vi "multi-function-fpga.vi"() -> ()   [LabVIEW 2016]
uses:
  <vilib>/rvi/Emulation/niFpgaGetClockAttributes.vi
  <vilib>/rvi/Emulation/niFpgaSctlEmulationGetInTimedLoop.vi
  <vilib>/rvi/Emulation/niFpgaEmulationReportErrorSimple.vi
  <vilib>/rvi/eio/common/nirviEmuTemplateMethod_errors.vi
  <vilib>/rvi/Emulation/niFpgaCriticalErrorInLSC.vi
  <vilib>/eio/EIONode/EIONode.xnode
panel:
  in  "and1":fxp<+/-,20,5>=3.5 format="%#_17g"
  in  "or15":fxp<+/-,20,5>=3.5 format="%#_17g"
  in  "or14":fxp<+/-,20,5>=3.5 format="%#_17g"
  in  "or13":fxp<+/-,20,5>=3.5 format="%#_17g"
  in  "or12":fxp<+/-,20,5>=3.5 format="%#_17g"
  in  "or11":fxp<+/-,20,5>=3.5 format="%#_17g"
  in  "or10":fxp<+/-,20,5>=3.5 format="%#_17g"
  in  "or9":fxp<+/-,20,5>=3.5 format="%#_17g"
  in  "or8":fxp<+/-,20,5>=3.5 format="%#_17g"
  in  "or7":fxp<+/-,20,5>=3.5 format="%#_17g"
  in  "or6":fxp<+/-,20,5>=3.5 format="%#_17g"
  in  "or5":fxp<+/-,20,5>=3.5 format="%#_17g"
  in  "or4":fxp<+/-,20,5>=3.5 format="%#_17g"
  in  "or3":fxp<+/-,20,5>=3.5 format="%#_17g"
  in  "or2":fxp<+/-,20,5>=3.5 format="%#_17g"
  in  "or1":fxp<+/-,20,5>=3.5 format="%#_17g"
  in  "or0":fxp<+/-,20,5>=3.5 format="%#_17g"
  in  "and15":fxp<+/-,20,5>=3.5 format="%#_17g"
  in  "and14":fxp<+/-,20,5>=3.5 format="%#_17g"
  in  "and13":fxp<+/-,20,5>=3.5 format="%#_17g"
  in  "and12":fxp<+/-,20,5>=3.5 format="%#_17g"
  in  "and11":fxp<+/-,20,5>=3.5 format="%#_17g"
  in  "and10":fxp<+/-,20,5>=3.5 format="%#_17g"
  in  "and9":fxp<+/-,20,5>=3.5 format="%#_17g"
  in  "and8":fxp<+/-,20,5>=3.5 format="%#_17g"
  in  "and7":fxp<+/-,20,5>=3.5 format="%#_17g"
  in  "and6":fxp<+/-,20,5>=3.5 format="%#_17g"
  in  "and5":fxp<+/-,20,5>=3.5 format="%#_17g"
  in  "and4":fxp<+/-,20,5>=3.5 format="%#_17g"
  in  "and3":fxp<+/-,20,5>=3.5 format="%#_17g"
  in  "and2":fxp<+/-,20,5>=3.5 format="%#_17g"
  in  "and0":fxp<+/-,20,5>=3.5 format="%#_17g"
  in  "s15":fxp<+/-,20,5>=3.5 format="%#_17g"
  in  "s14":fxp<+/-,20,5>=3.5 format="%#_17g"
  in  "s13":fxp<+/-,20,5>=3.5 format="%#_17g"
  in  "s12":fxp<+/-,20,5>=3.5 format="%#_17g"
  in  "s11":fxp<+/-,20,5>=3.5 format="%#_17g"
  in  "s10":fxp<+/-,20,5>=3.5 format="%#_17g"
  in  "s9":fxp<+/-,20,5>=3.5 format="%#_17g"
  in  "s8":fxp<+/-,20,5>=3.5 format="%#_17g"
  in  "s7":fxp<+/-,20,5>=3.5 format="%#_17g"
  in  "s6":fxp<+/-,20,5>=3.5 format="%#_17g"
  in  "s5":fxp<+/-,20,5>=3.5 format="%#_17g"
  in  "s4":fxp<+/-,20,5>=3.5 format="%#_17g"
  in  "s3":fxp<+/-,20,5>=3.5 format="%#_17g"
  in  "s2":fxp<+/-,20,5>=3.5 format="%#_17g"
  in  "s1":fxp<+/-,20,5>=3.5 format="%#_17g"
  in  "s0":fxp<+/-,20,5>=3.5 format="%#_17g"
  out "Mod2/DIO24":bool
  in  "OUT12":T1(ring)
  in  "iter12":fxp<+/-,20,5> format="%#_17g"
  out "Mod2/DIO26":bool
  in  "OUT13":T1(ring)
  in  "iter13":fxp<+/-,20,5> format="%#_17g"
  out "Mod2/DIO28":bool
  in  "OUT14":T1(ring)
  in  "iter14":fxp<+/-,20,5> format="%#_17g"
  out "Mod2/DIO30":bool
  in  "OUT15":T1(ring)
  in  "iter15":fxp<+/-,20,5> format="%#_17g"
  out "Mod2/DIO16":bool
  in  "OUT8":T1(ring)
  in  "iter8":fxp<+/-,20,5> format="%#_17g"
  out "Mod2/DIO18":bool
  in  "OUT9":T1(ring)
  in  "iter9":fxp<+/-,20,5> format="%#_17g"
  out "Mod2/DIO20":bool
  in  "OUT10":T1(ring)
  in  "iter10":fxp<+/-,20,5> format="%#_17g"
  out "Mod2/DIO22":bool
  in  "OUT11":T1(ring)
  in  "iter11":fxp<+/-,20,5> format="%#_17g"
  out "Mod2/DIO8":bool
  in  "OUT4":T1(ring)
  in  "iter4":fxp<+/-,20,5> format="%#_17g"
  out "Mod2/DIO10":bool
  in  "OUT5":T1(ring)
  in  "iter5":fxp<+/-,20,5> format="%#_17g"
  out "Mod2/DIO12":bool
  in  "OUT6":T1(ring)
  in  "iter6":fxp<+/-,20,5> format="%#_17g"
  out "Mod2/DIO14":bool
  in  "OUT7":T1(ring)
  in  "iter7":fxp<+/-,20,5> format="%#_17g"
  out "Mod2/DIO0":bool
  in  "OUT0":T1(ring)
  in  "iter0":fxp<+/-,20,5> format="%#_17g"
  out "Mod2/DIO2":bool
  in  "OUT1":T1(ring)
  in  "iter1":fxp<+/-,20,5> format="%#_17g"
  out "Mod2/DIO4":bool
  in  "OUT2":T1(ring)
  in  "iter2":fxp<+/-,20,5> format="%#_17g"
  out "Mod2/DIO6":bool
  in  "iter3":fxp<+/-,20,5> format="%#_17g"
  in  "OUT3":T1(ring)
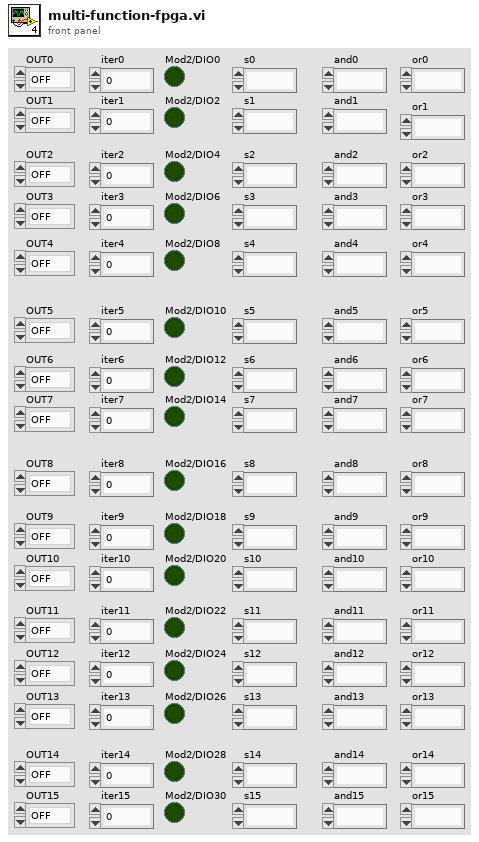
[diagram p1: front panel]
types:
  T1 = enum16{"OFF", "SWITCH", "AND GATE", "OR GATE", "ITERATION"}
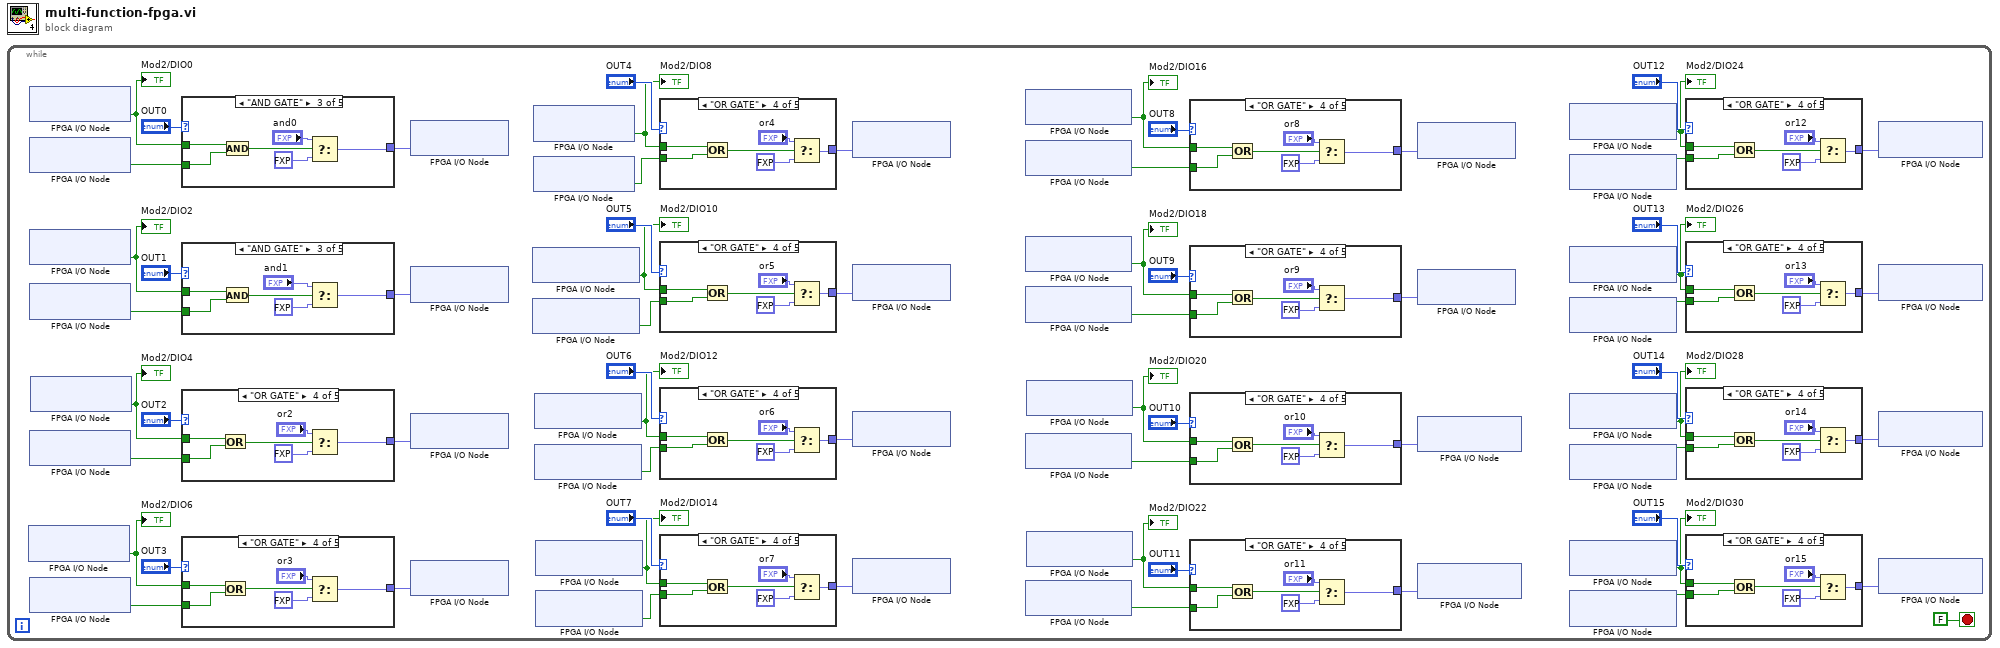
[diagram p0: block diagram]
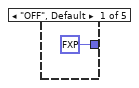
[diagram p2: hidden frame]
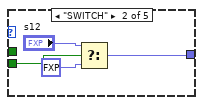
[diagram p3: hidden frame]
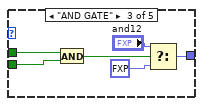
[diagram p4: hidden frame]
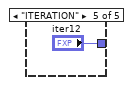
[diagram p5: hidden frame]
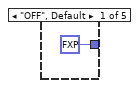
[diagram p6: hidden frame]
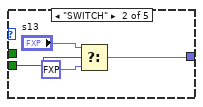
[diagram p7: hidden frame]
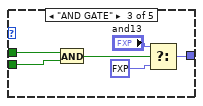
[diagram p8: hidden frame]
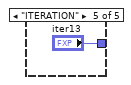
[diagram p9: hidden frame]
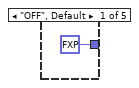
[diagram p10: hidden frame]
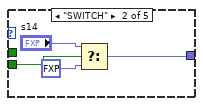
[diagram p11: hidden frame]
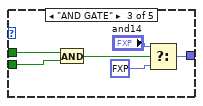
[diagram p12: hidden frame]
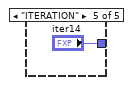
[diagram p13: hidden frame]
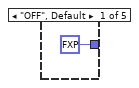
[diagram p14: hidden frame]
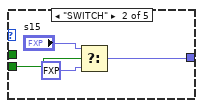
[diagram p15: hidden frame]
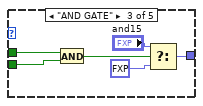
[diagram p16: hidden frame]
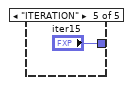
[diagram p17: hidden frame]
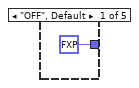
[diagram p18: hidden frame]
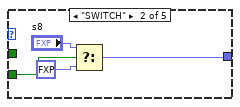
[diagram p19: hidden frame]
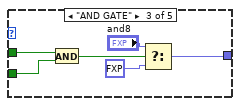
[diagram p20: hidden frame]
diagram:
  n1 = while {
    stop <- FALSE stop-if-true
    n2 = xnode "FPGA I/O Node"() -> ("Mod2/DIO6"=w62:bool)  [unwired: 1 in, 1 out]
    "Mod2/DIO6" <- w62
    n3 = xnode "FPGA I/O Node"() -> ("Mod2/DIO0"=w50:bool)  [unwired: 1 in, 1 out]
    "Mod2/DIO0" <- w50
    n4 = xnode "FPGA I/O Node"() -> ("Mod2/DIO1"=w51:bool)  [unwired: 1 in, 1 out]
    n5 = xnode "FPGA I/O Node"() -> ("Mod2/DIO2"=w54:bool)  [unwired: 1 in, 1 out]
    "Mod2/DIO2" <- w54
    n6 = xnode "FPGA I/O Node"() -> ("Mod2/DIO3"=w55:bool)  [unwired: 1 in, 1 out]
    n7 = xnode "FPGA I/O Node"() -> ("Mod2/DIO5"=w59:bool)  [unwired: 1 in, 1 out]
    n8 = xnode "FPGA I/O Node"() -> ("Mod2/DIO7"=w64:bool)  [unwired: 1 in, 1 out]
    n9 = xnode "FPGA I/O Node"() -> ("Mod2/DIO4"=w58:bool)  [unwired: 1 in, 1 out]
    "Mod2/DIO4" <- w58
    n10 = case shown="\"AND GATE\"" "OUT0" {
      tunnel: w51 -> [_ w286 w291 w297 _]
      tunnel: w50 -> [_ _ w292 w298 _]
      tunnel: [fxp<+/-,20,5> 0.0 ("Mod4/AO0") w283 w287 w293 "iter0"] -> w49
      frame "OFF", Default {
      }
      frame "SWITCH" {
        n11 = Select(t="s0", s=w286, f=fxp<+/-,20,5> 0.0 ("Mod4/AO0")) -> (s? t:f=w283:fxp<+/-,20,5>)
      }
      frame "AND GATE" {
        n12 = And(x=w292, y=w291) -> (x .and. y?=w288:bool)
        n13 = Select(t="and0", s=w288, f=fxp<+/-,20,5> 0.0 ("Mod4/AO0")) -> (s? t:f=w287:fxp<+/-,20,5>)
      }
      frame "OR GATE" {
        n14 = Or(x=w298, y=w297) -> (x .or. y?=w296:bool)
        n15 = Select(t="or0", s=w296, f=fxp<+/-,20,5> 0.0 ("Mod4/AO0")) -> (s? t:f=w293:fxp<+/-,20,5>)
      }
      frame "ITERATION" {
      }
    }
    n16 = case shown="\"AND GATE\"" "OUT1" {
      tunnel: w55 -> [_ w304 w309 w315 _]
      tunnel: w54 -> [_ _ w310 w316 _]
      tunnel: [fxp<+/-,20,5> 0.0 ("Mod4/AO0") w301 w305 w311 "iter1"] -> w53
      frame "OFF", Default {
      }
      frame "SWITCH" {
        n17 = Select(t="s1", s=w304, f=fxp<+/-,20,5> 0.0 ("Mod4/AO0")) -> (s? t:f=w301:fxp<+/-,20,5>)
      }
      frame "AND GATE" {
        n18 = And(x=w310, y=w309) -> (x .and. y?=w306:bool)
        n19 = Select(t="and1", s=w306, f=fxp<+/-,20,5> 0.0 ("Mod4/AO0")) -> (s? t:f=w305:fxp<+/-,20,5>)
      }
      frame "OR GATE" {
        n20 = Or(x=w316, y=w315) -> (x .or. y?=w314:bool)
        n21 = Select(t="or1", s=w314, f=fxp<+/-,20,5> 0.0 ("Mod4/AO0")) -> (s? t:f=w311:fxp<+/-,20,5>)
      }
      frame "ITERATION" {
      }
    }
    n22 = case shown="\"OR GATE\"" "OUT2" {
      tunnel: w59 -> [_ w322 w327 w333 _]
      tunnel: w58 -> [_ _ w328 w334 _]
      tunnel: [fxp<+/-,20,5> 0.0 ("Mod4/AO0") w319 w323 w329 "iter2"] -> w57
      frame "OFF", Default {
      }
      frame "SWITCH" {
        n23 = Select(t="s2", s=w322, f=fxp<+/-,20,5> 0.0 ("Mod4/AO0")) -> (s? t:f=w319:fxp<+/-,20,5>)
      }
      frame "AND GATE" {
        n24 = And(x=w328, y=w327) -> (x .and. y?=w324:bool)
        n25 = Select(t="and2", s=w324, f=fxp<+/-,20,5> 0.0 ("Mod4/AO0")) -> (s? t:f=w323:fxp<+/-,20,5>)
      }
      frame "OR GATE" {
        n26 = Or(x=w334, y=w333) -> (x .or. y?=w332:bool)
        n27 = Select(t="or2", s=w332, f=fxp<+/-,20,5> 0.0 ("Mod4/AO0")) -> (s? t:f=w329:fxp<+/-,20,5>)
      }
      frame "ITERATION" {
      }
    }
    n28 = case shown="\"OR GATE\"" "OUT3" {
      tunnel: w64 -> [_ w340 w345 w351 _]
      tunnel: w62 -> [_ _ w346 w352 _]
      tunnel: [fxp<+/-,20,5> 0.0 ("Mod4/AO0") w337 w341 w347 "iter3"] -> w61
      frame "OFF", Default {
      }
      frame "SWITCH" {
        n29 = Select(t="s3", s=w340, f=fxp<+/-,20,5> 0.0 ("Mod4/AO0")) -> (s? t:f=w337:fxp<+/-,20,5>)
      }
      frame "AND GATE" {
        n30 = And(x=w346, y=w345) -> (x .and. y?=w342:bool)
        n31 = Select(t="and3", s=w342, f=fxp<+/-,20,5> 0.0 ("Mod4/AO0")) -> (s? t:f=w341:fxp<+/-,20,5>)
      }
      frame "OR GATE" {
        n32 = Or(x=w352, y=w351) -> (x .or. y?=w350:bool)
        n33 = Select(t="or3", s=w350, f=fxp<+/-,20,5> 0.0 ("Mod4/AO0")) -> (s? t:f=w347:fxp<+/-,20,5>)
      }
      frame "ITERATION" {
      }
    }
    n34 = xnode "FPGA I/O Node"("Mod4/AO0"=w49) -> ()  [unwired: 1 in, 1 out]
    n35 = xnode "FPGA I/O Node"("Mod4/AO1"=w53) -> ()  [unwired: 1 in, 1 out]
    n36 = xnode "FPGA I/O Node"("Mod4/AO2"=w57) -> ()  [unwired: 1 in, 1 out]
    n37 = xnode "FPGA I/O Node"("Mod4/AO3"=w61) -> ()  [unwired: 1 in, 1 out]
    n38 = xnode "FPGA I/O Node"() -> ("Mod2/DIO10"=w38:bool)  [unwired: 1 in, 1 out]
    "Mod2/DIO10" <- w38
    n39 = xnode "FPGA I/O Node"() -> ("Mod2/DIO11"=w39:bool)  [unwired: 1 in, 1 out]
    n40 = xnode "FPGA I/O Node"() -> ("Mod2/DIO8"=w34:bool)  [unwired: 1 in, 1 out]
    "Mod2/DIO8" <- w34
    n41 = xnode "FPGA I/O Node"() -> ("Mod2/DIO9"=w35:bool)  [unwired: 1 in, 1 out]
    n42 = xnode "FPGA I/O Node"() -> ("Mod2/DIO12"=w42:bool)  [unwired: 1 in, 1 out]
    "Mod2/DIO12" <- w42
    n43 = xnode "FPGA I/O Node"() -> ("Mod2/DIO13"=w43:bool)  [unwired: 1 in, 1 out]
    n44 = xnode "FPGA I/O Node"() -> ("Mod2/DIO14"=w46:bool)  [unwired: 1 in, 1 out]
    "Mod2/DIO14" <- w46
    n45 = xnode "FPGA I/O Node"() -> ("Mod2/DIO15"=w47:bool)  [unwired: 1 in, 1 out]
    n46 = case shown="\"OR GATE\"" "OUT4" {
      tunnel: w35 -> [_ w214 w219 w225 _]
      tunnel: w34 -> [_ _ w220 w226 _]
      tunnel: [fxp<+/-,20,5> 0.0 ("Mod4/AO0") w211 w215 w221 "iter4"] -> w33
      frame "OFF", Default {
      }
      frame "SWITCH" {
        n47 = Select(t="s4", s=w214, f=fxp<+/-,20,5> 0.0 ("Mod4/AO0")) -> (s? t:f=w211:fxp<+/-,20,5>)
      }
      frame "AND GATE" {
        n48 = And(x=w220, y=w219) -> (x .and. y?=w216:bool)
        n49 = Select(t="and4", s=w216, f=fxp<+/-,20,5> 0.0 ("Mod4/AO0")) -> (s? t:f=w215:fxp<+/-,20,5>)
      }
      frame "OR GATE" {
        n50 = Or(x=w226, y=w225) -> (x .or. y?=w224:bool)
        n51 = Select(t="or4", s=w224, f=fxp<+/-,20,5> 0.0 ("Mod4/AO0")) -> (s? t:f=w221:fxp<+/-,20,5>)
      }
      frame "ITERATION" {
      }
    }
    n52 = case shown="\"OR GATE\"" "OUT5" {
      tunnel: w39 -> [_ w232 w237 w243 _]
      tunnel: w38 -> [_ _ w238 w244 _]
      tunnel: [fxp<+/-,20,5> 0.0 ("Mod4/AO0") w229 w233 w239 "iter5"] -> w37
      frame "OFF", Default {
      }
      frame "SWITCH" {
        n53 = Select(t="s5", s=w232, f=fxp<+/-,20,5> 0.0 ("Mod4/AO0")) -> (s? t:f=w229:fxp<+/-,20,5>)
      }
      frame "AND GATE" {
        n54 = And(x=w238, y=w237) -> (x .and. y?=w234:bool)
        n55 = Select(t="and5", s=w234, f=fxp<+/-,20,5> 0.0 ("Mod4/AO0")) -> (s? t:f=w233:fxp<+/-,20,5>)
      }
      frame "OR GATE" {
        n56 = Or(x=w244, y=w243) -> (x .or. y?=w242:bool)
        n57 = Select(t="or5", s=w242, f=fxp<+/-,20,5> 0.0 ("Mod4/AO0")) -> (s? t:f=w239:fxp<+/-,20,5>)
      }
      frame "ITERATION" {
      }
    }
    n58 = case shown="\"OR GATE\"" "OUT6" {
      tunnel: w43 -> [_ w250 w255 w261 _]
      tunnel: w42 -> [_ _ w256 w262 _]
      tunnel: [fxp<+/-,20,5> 0.0 ("Mod4/AO0") w247 w251 w257 "iter6"] -> w41
      frame "OFF", Default {
      }
      frame "SWITCH" {
        n59 = Select(t="s6", s=w250, f=fxp<+/-,20,5> 0.0 ("Mod4/AO0")) -> (s? t:f=w247:fxp<+/-,20,5>)
      }
      frame "AND GATE" {
        n60 = And(x=w256, y=w255) -> (x .and. y?=w252:bool)
        n61 = Select(t="and6", s=w252, f=fxp<+/-,20,5> 0.0 ("Mod4/AO0")) -> (s? t:f=w251:fxp<+/-,20,5>)
      }
      frame "OR GATE" {
        n62 = Or(x=w262, y=w261) -> (x .or. y?=w260:bool)
        n63 = Select(t="or6", s=w260, f=fxp<+/-,20,5> 0.0 ("Mod4/AO0")) -> (s? t:f=w257:fxp<+/-,20,5>)
      }
      frame "ITERATION" {
      }
    }
    n64 = case shown="\"OR GATE\"" "OUT7" {
      tunnel: w47 -> [_ w268 w273 w279 _]
      tunnel: w46 -> [_ _ w274 w280 _]
      tunnel: [fxp<+/-,20,5> 0.0 ("Mod4/AO0") w265 w269 w275 "iter7"] -> w45
      frame "OFF", Default {
      }
      frame "SWITCH" {
        n65 = Select(t="s7", s=w268, f=fxp<+/-,20,5> 0.0 ("Mod4/AO0")) -> (s? t:f=w265:fxp<+/-,20,5>)
      }
      frame "AND GATE" {
        n66 = And(x=w274, y=w273) -> (x .and. y?=w270:bool)
        n67 = Select(t="and7", s=w270, f=fxp<+/-,20,5> 0.0 ("Mod4/AO0")) -> (s? t:f=w269:fxp<+/-,20,5>)
      }
      frame "OR GATE" {
        n68 = Or(x=w280, y=w279) -> (x .or. y?=w278:bool)
        n69 = Select(t="or7", s=w278, f=fxp<+/-,20,5> 0.0 ("Mod4/AO0")) -> (s? t:f=w275:fxp<+/-,20,5>)
      }
      frame "ITERATION" {
      }
    }
    n70 = xnode "FPGA I/O Node"("Mod4/AO4"=w33) -> ()  [unwired: 1 in, 1 out]
    n71 = xnode "FPGA I/O Node"("Mod4/AO5"=w37) -> ()  [unwired: 1 in, 1 out]
    n72 = xnode "FPGA I/O Node"("Mod4/AO6"=w41) -> ()  [unwired: 1 in, 1 out]
    n73 = xnode "FPGA I/O Node"("Mod4/AO7"=w45) -> ()  [unwired: 1 in, 1 out]
    n74 = xnode "FPGA I/O Node"() -> ("Mod2/DIO16"=w18:bool)  [unwired: 1 in, 1 out]
    "Mod2/DIO16" <- w18
    n75 = xnode "FPGA I/O Node"() -> ("Mod2/DIO17"=w19:bool)  [unwired: 1 in, 1 out]
    n76 = xnode "FPGA I/O Node"() -> ("Mod2/DIO18"=w22:bool)  [unwired: 1 in, 1 out]
    "Mod2/DIO18" <- w22
    n77 = xnode "FPGA I/O Node"() -> ("Mod2/DIO19"=w23:bool)  [unwired: 1 in, 1 out]
    n78 = xnode "FPGA I/O Node"() -> ("Mod2/DIO21"=w27:bool)  [unwired: 1 in, 1 out]
    n79 = xnode "FPGA I/O Node"() -> ("Mod2/DIO23"=w31:bool)  [unwired: 1 in, 1 out]
    n80 = xnode "FPGA I/O Node"() -> ("Mod2/DIO20"=w26:bool)  [unwired: 1 in, 1 out]
    "Mod2/DIO20" <- w26
    n81 = xnode "FPGA I/O Node"() -> ("Mod2/DIO22"=w30:bool)  [unwired: 1 in, 1 out]
    "Mod2/DIO22" <- w30
    n82 = case shown="\"OR GATE\"" "OUT8" {
      tunnel: w19 -> [_ w142 w147 w153 _]
      tunnel: w18 -> [_ _ w148 w154 _]
      tunnel: [fxp<+/-,20,5> 0.0 ("Mod4/AO0") w139 w143 w149 "iter8"] -> w17
      frame "OFF", Default {
      }
      frame "SWITCH" {
        n83 = Select(t="s8", s=w142, f=fxp<+/-,20,5> 0.0 ("Mod4/AO0")) -> (s? t:f=w139:fxp<+/-,20,5>)
      }
      frame "AND GATE" {
        n84 = And(x=w148, y=w147) -> (x .and. y?=w144:bool)
        n85 = Select(t="and8", s=w144, f=fxp<+/-,20,5> 0.0 ("Mod4/AO0")) -> (s? t:f=w143:fxp<+/-,20,5>)
      }
      frame "OR GATE" {
        n86 = Or(x=w154, y=w153) -> (x .or. y?=w152:bool)
        n87 = Select(t="or8", s=w152, f=fxp<+/-,20,5> 0.0 ("Mod4/AO0")) -> (s? t:f=w149:fxp<+/-,20,5>)
      }
      frame "ITERATION" {
      }
    }
    n88 = case shown="\"OR GATE\"" "OUT9" {
      tunnel: w23 -> [_ w160 w165 w171 _]
      tunnel: w22 -> [_ _ w166 w172 _]
      tunnel: [fxp<+/-,20,5> 0.0 ("Mod4/AO0") w157 w161 w167 "iter9"] -> w21
      frame "OFF", Default {
      }
      frame "SWITCH" {
        n89 = Select(t="s9", s=w160, f=fxp<+/-,20,5> 0.0 ("Mod4/AO0")) -> (s? t:f=w157:fxp<+/-,20,5>)
      }
      frame "AND GATE" {
        n90 = And(x=w166, y=w165) -> (x .and. y?=w162:bool)
        n91 = Select(t="and9", s=w162, f=fxp<+/-,20,5> 0.0 ("Mod4/AO0")) -> (s? t:f=w161:fxp<+/-,20,5>)
      }
      frame "OR GATE" {
        n92 = Or(x=w172, y=w171) -> (x .or. y?=w170:bool)
        n93 = Select(t="or9", s=w170, f=fxp<+/-,20,5> 0.0 ("Mod4/AO0")) -> (s? t:f=w167:fxp<+/-,20,5>)
      }
      frame "ITERATION" {
      }
    }
    n94 = case shown="\"OR GATE\"" "OUT10" {
      tunnel: w27 -> [_ w178 w183 w189 _]
      tunnel: w26 -> [_ _ w184 w190 _]
      tunnel: [fxp<+/-,20,5> 0.0 ("Mod4/AO0") w175 w179 w185 "iter10"] -> w25
      frame "OFF", Default {
      }
      frame "SWITCH" {
        n95 = Select(t="s10", s=w178, f=fxp<+/-,20,5> 0.0 ("Mod4/AO0")) -> (s? t:f=w175:fxp<+/-,20,5>)
      }
      frame "AND GATE" {
        n96 = And(x=w184, y=w183) -> (x .and. y?=w180:bool)
        n97 = Select(t="and10", s=w180, f=fxp<+/-,20,5> 0.0 ("Mod4/AO0")) -> (s? t:f=w179:fxp<+/-,20,5>)
      }
      frame "OR GATE" {
        n98 = Or(x=w190, y=w189) -> (x .or. y?=w188:bool)
        n99 = Select(t="or10", s=w188, f=fxp<+/-,20,5> 0.0 ("Mod4/AO0")) -> (s? t:f=w185:fxp<+/-,20,5>)
      }
      frame "ITERATION" {
      }
    }
    n100 = case shown="\"OR GATE\"" "OUT11" {
      tunnel: w31 -> [_ w196 w201 w207 _]
      tunnel: w30 -> [_ _ w202 w208 _]
      tunnel: [fxp<+/-,20,5> 0.0 ("Mod4/AO0") w193 w197 w203 "iter11"] -> w29
      frame "OFF", Default {
      }
      frame "SWITCH" {
        n101 = Select(t="s11", s=w196, f=fxp<+/-,20,5> 0.0 ("Mod4/AO0")) -> (s? t:f=w193:fxp<+/-,20,5>)
      }
      frame "AND GATE" {
        n102 = And(x=w202, y=w201) -> (x .and. y?=w198:bool)
        n103 = Select(t="and11", s=w198, f=fxp<+/-,20,5> 0.0 ("Mod4/AO0")) -> (s? t:f=w197:fxp<+/-,20,5>)
      }
      frame "OR GATE" {
        n104 = Or(x=w208, y=w207) -> (x .or. y?=w206:bool)
        n105 = Select(t="or11", s=w206, f=fxp<+/-,20,5> 0.0 ("Mod4/AO0")) -> (s? t:f=w203:fxp<+/-,20,5>)
      }
      frame "ITERATION" {
      }
    }
    n106 = xnode "FPGA I/O Node"("Mod4/AO8"=w17) -> ()  [unwired: 1 in, 1 out]
    n107 = xnode "FPGA I/O Node"("Mod4/AO9"=w21) -> ()  [unwired: 1 in, 1 out]
    n108 = xnode "FPGA I/O Node"("Mod4/AO10"=w25) -> ()  [unwired: 1 in, 1 out]
    n109 = xnode "FPGA I/O Node"("Mod4/AO11"=w29) -> ()  [unwired: 1 in, 1 out]
    n110 = xnode "FPGA I/O Node"() -> ("Mod2/DIO24"=w2:bool)  [unwired: 1 in, 1 out]
    "Mod2/DIO24" <- w2
    n111 = xnode "FPGA I/O Node"() -> ("Mod2/DIO25"=w3:bool)  [unwired: 1 in, 1 out]
    n112 = xnode "FPGA I/O Node"() -> ("Mod2/DIO26"=w6:bool)  [unwired: 1 in, 1 out]
    "Mod2/DIO26" <- w6
    n113 = xnode "FPGA I/O Node"() -> ("Mod2/DIO27"=w7:bool)  [unwired: 1 in, 1 out]
    n114 = xnode "FPGA I/O Node"() -> ("Mod2/DIO28"=w10:bool)  [unwired: 1 in, 1 out]
    "Mod2/DIO28" <- w10
    n115 = xnode "FPGA I/O Node"() -> ("Mod2/DIO29"=w11:bool)  [unwired: 1 in, 1 out]
    n116 = xnode "FPGA I/O Node"() -> ("Mod2/DIO30"=w14:bool)  [unwired: 1 in, 1 out]
    "Mod2/DIO30" <- w14
    n117 = xnode "FPGA I/O Node"() -> ("Mod2/DIO31"=w15:bool)  [unwired: 1 in, 1 out]
    n118 = case shown="\"OR GATE\"" "OUT12" {
      tunnel: w3 -> [_ w70 w75 w81 _]
      tunnel: w2 -> [_ _ w76 w82 _]
      tunnel: [fxp<+/-,20,5> 0.0 ("Mod4/AO0") w67 w71 w77 "iter12"] -> w1
      frame "OFF", Default {
      }
      frame "SWITCH" {
        n119 = Select(t="s12", s=w70, f=fxp<+/-,20,5> 0.0 ("Mod4/AO0")) -> (s? t:f=w67:fxp<+/-,20,5>)
      }
      frame "AND GATE" {
        n120 = And(x=w76, y=w75) -> (x .and. y?=w72:bool)
        n121 = Select(t="and12", s=w72, f=fxp<+/-,20,5> 0.0 ("Mod4/AO0")) -> (s? t:f=w71:fxp<+/-,20,5>)
      }
      frame "OR GATE" {
        n122 = Or(x=w82, y=w81) -> (x .or. y?=w80:bool)
        n123 = Select(t="or12", s=w80, f=fxp<+/-,20,5> 0.0 ("Mod4/AO0")) -> (s? t:f=w77:fxp<+/-,20,5>)
      }
      frame "ITERATION" {
      }
    }
    n124 = case shown="\"OR GATE\"" "OUT13" {
      tunnel: w7 -> [_ w88 w93 w99 _]
      tunnel: w6 -> [_ _ w94 w100 _]
      tunnel: [fxp<+/-,20,5> 0.0 ("Mod4/AO0") w85 w89 w95 "iter13"] -> w5
      frame "OFF", Default {
      }
      frame "SWITCH" {
        n125 = Select(t="s13", s=w88, f=fxp<+/-,20,5> 0.0 ("Mod4/AO0")) -> (s? t:f=w85:fxp<+/-,20,5>)
      }
      frame "AND GATE" {
        n126 = And(x=w94, y=w93) -> (x .and. y?=w90:bool)
        n127 = Select(t="and13", s=w90, f=fxp<+/-,20,5> 0.0 ("Mod4/AO0")) -> (s? t:f=w89:fxp<+/-,20,5>)
      }
      frame "OR GATE" {
        n128 = Or(x=w100, y=w99) -> (x .or. y?=w98:bool)
        n129 = Select(t="or13", s=w98, f=fxp<+/-,20,5> 0.0 ("Mod4/AO0")) -> (s? t:f=w95:fxp<+/-,20,5>)
      }
      frame "ITERATION" {
      }
    }
    n130 = case shown="\"OR GATE\"" "OUT14" {
      tunnel: w11 -> [_ w106 w111 w117 _]
      tunnel: w10 -> [_ _ w112 w118 _]
      tunnel: [fxp<+/-,20,5> 0.0 ("Mod4/AO0") w103 w107 w113 "iter14"] -> w9
      frame "OFF", Default {
      }
      frame "SWITCH" {
        n131 = Select(t="s14", s=w106, f=fxp<+/-,20,5> 0.0 ("Mod4/AO0")) -> (s? t:f=w103:fxp<+/-,20,5>)
      }
      frame "AND GATE" {
        n132 = And(x=w112, y=w111) -> (x .and. y?=w108:bool)
        n133 = Select(t="and14", s=w108, f=fxp<+/-,20,5> 0.0 ("Mod4/AO0")) -> (s? t:f=w107:fxp<+/-,20,5>)
      }
      frame "OR GATE" {
        n134 = Or(x=w118, y=w117) -> (x .or. y?=w116:bool)
        n135 = Select(t="or14", s=w116, f=fxp<+/-,20,5> 0.0 ("Mod4/AO0")) -> (s? t:f=w113:fxp<+/-,20,5>)
      }
      frame "ITERATION" {
      }
    }
    n136 = case shown="\"OR GATE\"" "OUT15" {
      tunnel: w15 -> [_ w124 w129 w135 _]
      tunnel: w14 -> [_ _ w130 w136 _]
      tunnel: [fxp<+/-,20,5> 0.0 ("Mod4/AO0") w121 w125 w131 "iter15"] -> w13
      frame "OFF", Default {
      }
      frame "SWITCH" {
        n137 = Select(t="s15", s=w124, f=fxp<+/-,20,5> 0.0 ("Mod4/AO0")) -> (s? t:f=w121:fxp<+/-,20,5>)
      }
      frame "AND GATE" {
        n138 = And(x=w130, y=w129) -> (x .and. y?=w126:bool)
        n139 = Select(t="and15", s=w126, f=fxp<+/-,20,5> 0.0 ("Mod4/AO0")) -> (s? t:f=w125:fxp<+/-,20,5>)
      }
      frame "OR GATE" {
        n140 = Or(x=w136, y=w135) -> (x .or. y?=w134:bool)
        n141 = Select(t="or15", s=w134, f=fxp<+/-,20,5> 0.0 ("Mod4/AO0")) -> (s? t:f=w131:fxp<+/-,20,5>)
      }
      frame "ITERATION" {
      }
    }
    n142 = xnode "FPGA I/O Node"("Mod4/AO12"=w1) -> ()  [unwired: 1 in, 1 out]
    n143 = xnode "FPGA I/O Node"("Mod4/AO13"=w5) -> ()  [unwired: 1 in, 1 out]
    n144 = xnode "FPGA I/O Node"("Mod4/AO14"=w9) -> ()  [unwired: 1 in, 1 out]
    n145 = xnode "FPGA I/O Node"("Mod4/AO15"=w13) -> ()  [unwired: 1 in, 1 out]
  }
